vi "Window control.vi"(5 "error in (no error)":errorcluster) -> (19 "error out":errorcluster)   [LabVIEW 2010]
doc: "This VI is used to check if the VI/Window was closed by the user.\n\nTRUE if the caller window/VI is closed.\nFALSE if the caller winwow/VI is still open.\n\n------------------------------------------------------------------------------------------------------\nversion 1.0 by Donald Heyman CIT Engineering NV"
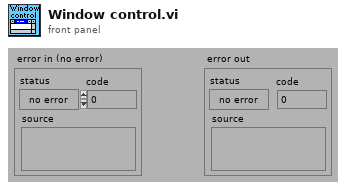
[diagram p1: front panel]
types:
  T1 = enum32{"invalid app kind", "Development System", "Run Time System", "Student Edition", "Embedded LabVIEW", "Evaluation", "Custom"}
  T2 = enum32{"Invalid", "Default", "Floating", "Floating/Auto-Hide", "Modal"}
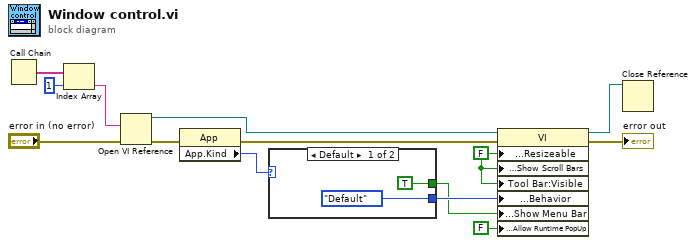
[diagram p0: block diagram]
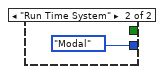
[diagram p2: hidden frame]
diagram:
  w1 = FALSE ("Front Panel Window:Resizable")
  n1 = Call Chain() -> (call chain=w14:string[])
  n2 = Index Array(array=w14, index=1) -> (element=w11:string)
  n3 = Open VI Reference(vi path=w11, error in (no error)="error in (no error)") -> (vi reference=w10:refnum<vi>, error out=w9:errorcluster)  [unwired: 4 in]
  n4 = property class="App"(error in=w9) -> (error out=w6:errorcluster, "App.Kind"=w8:T1)  [unwired: 1 in, 1 out]
  n5 = case shown="Default" w8 {
    tunnel: [T2."Default" ("Front Panel Window:Behavior") T2."Modal" ("Front Panel Window:Behavior")] -> w7
    tunnel: [TRUE ("Front Panel Window:Show Scroll Bars") _] -> w2
    frame Default {
    }
    frame "Run Time System" {
    }
  }
  n6 = property class="VI"(reference=w10, error in=w6, "Front Panel Window:Resizeable"=w1, "Front Panel Window:Show Scroll Bars"=w1, "Tool Bar:Visible"=w1, "Front Panel Window:Behavior"=w7, "Front Panel Window:Show Menu Bar"=w2, "Front Panel Window:Allow Runtime PopUp"=FALSE) -> (reference out=w3:refnum<vi>, error out=→"error out":errorcluster)
  n7 = Close Reference(reference=w3) -> ()  [unwired: 1 in, 1 out]
